vi "Process Helper.vi"(7 "UI Ref":refnum<vi>, 10 "current time":timestamp, 11 "Settings in":T1) -> (0 "Digital Values to Write":bool[](array[boolean]), 1 "Analog Values to Write":dbl[](array[numeric]), 2 "Sequence State Channels to Write":dbl[](array[numeric]), 3 "Settings out":T1, 4 "New Settings":string, 5 "Changed":bool)   [LabVIEW 2020, in "Sequencer with Output Values.lvlib" / "Sequencer with Output Values.lvclass"]
uses:
  Sequencer with Output Values.lvclass
  Params.ctl
  Step Settings.ctl
  <vilib>/FlexLogger/SDK/PluginSDK.lvlibp
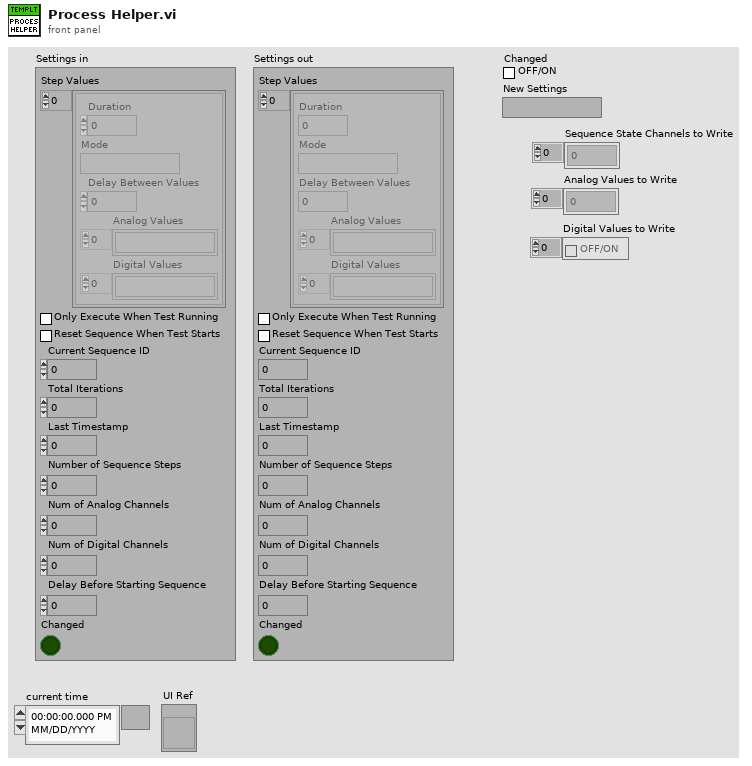
[diagram p1: front panel]
types:
  T1 = typedef "Sequencer with Output Values.lvlib/Sequencer with Output Values.lvclass/Params.ctl" = cluster{"Step Values":T2[], "Only Execute When Test Running":bool, "Reset Sequence When Test Starts":bool, "Current Sequence ID":u32, "Total Iterations":u32, "Last Timestamp":dbl, "Number of Sequence Steps":i32, "Num of Analog Channels":i32, "Num of Digital Channels":i32, "Delay Before Starting Sequence":dbl, "Changed":bool}
  T2 = typedef "Sequencer with Output Values.lvlib/Sequencer with Output Values.lvclass/Step Settings.ctl" = cluster{"Duration":dbl, "Mode":string, "Delay Between Values":dbl, "Analog Values":string[], "Digital Values":string[]}
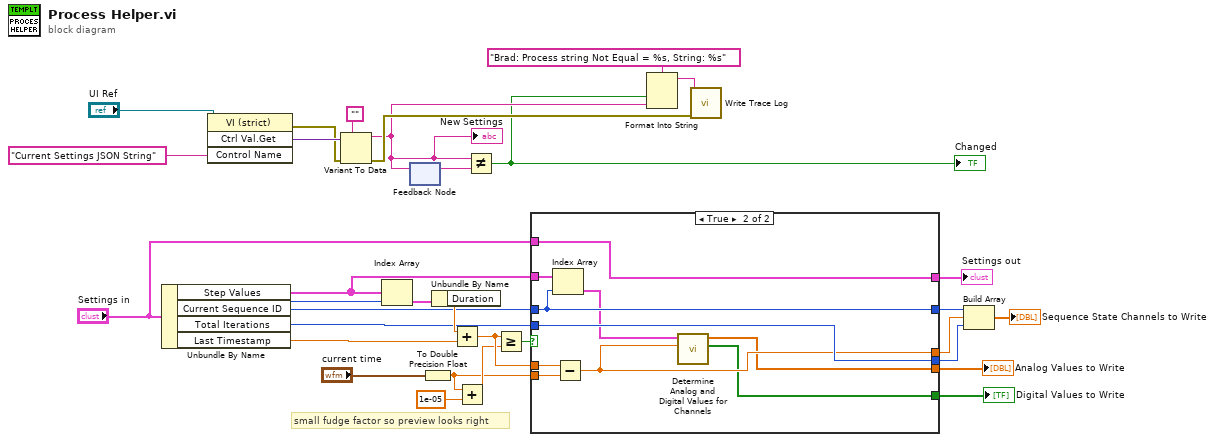
[diagram p0: block diagram]
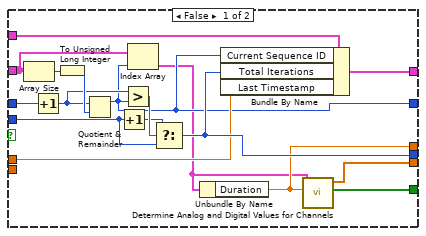
[diagram p2: hidden frame]
diagram:
  # "small fudge factor so preview looks right"
  n1 = Unbundle By Name("Settings in") -> ("Step Values"=w19:T2[], "Current Sequence ID"=w21:u32, "Total Iterations"=w20:u32, "Last Timestamp"=w23:dbl)
  n2 = invoke class="VI (strict)" method="Ctrl Val.Get"(reference="UI Ref", "Control Name"="Current Settings JSON String") -> (error out=w9:errorcluster, "Get Control Value Variant"=w10:variant)  [unwired: 2 in, 2 out]
  n3 = Variant To Data(error in=w9, type="", Variant=w10) -> (data=w4:string, error out=w5:errorcluster)
  "New Settings" <- w4
  n4 = Index Array(array=w19, index=w21) -> (element=w30:T2)
  n5 = feedback-in #1(w4) -> ()
  n6 = feedback #1() -> (w7:string)  [unwired: 1 in]
  n7 = To Double Precision Float(number="current time") -> (double precision float=w13:dbl)
  n8 = Unbundle By Name(w30) -> ("Duration"=w25:dbl)
  n9 = Add(x=w25, y=w23) -> (x+y=w27:dbl)
  n10 = Add(x=w13, y=1e-05) -> (x+y=w14:dbl)
  n11 = Not Equal?(x=w4, y=w7) -> (x != y?=w2:bool)
  "Changed" <- w2
  n12 = Greater Or Equal?(x=w27, y=w14) -> (x >= y?=w22:bool)
  n13 = case shown="True" w22 {
    tunnel: "Settings in" -> [w43 w57]
    tunnel: w21 -> [w47 w53]
    tunnel: w19 -> [w37 w54]
    tunnel: w20 -> [w45 w58]
    tunnel: [w36 w53] -> w24
    tunnel: [w41 w58] -> w26
    tunnel: [w42 w57] -> w31
    tunnel: w27 -> [w38 w56]
    tunnel: w13 -> [_ w55]
    tunnel: [w33 w51] -> w28
    tunnel: [w35 w50] -> w17
    tunnel: [w34 w49] -> w29
    frame False {
      n14 = Array Size(array=w37) -> (size(s)=w48:i32)
      n15 = Increment(x=w47) -> (x+1=w39:u32)
      n16 = To Unsigned Long Integer(number=w48) -> (unsigned 32bit integer=w40:u32)
      n17 = Quotient & Remainder(x=w39, y=w40) -> (x-y*floor(x/y)=w36:u32)  [unwired: 1 out]
      n18 = Increment(x=w45) -> (x+1=w44:u32)
      n19 = Greater?(x=w39, y=w36) -> (0:w46:bool)
      n20 = Index Array(array=w37, index=w36) -> (element=w32:T2)
      n21 = Select(t=w44, s=w46, f=w45) -> (s? t:f=w41:u32)
      n22 = Unbundle By Name(w32) -> ("Duration"=w33:dbl)
      n23 = Bundle By Name(cluster=w43, "Current Sequence ID"=w36, "Total Iterations"=w41, "Last Timestamp"=w38) -> (w42:T1)
      n24 = call "Determine Analog and Digital Values for Channels.vi"("Remaining Time"=w33, "Step Settings"=w32) -> ("Digital Values to Write"=w34:bool[], "Analog Values to Write"=w35:dbl[])  [unwired: 8 in]
    }
    frame True {
      n25 = Index Array(array=w54, index=w53) -> (element=w52:T2)
      n26 = Subtract(x=w56, y=w55) -> (x-y=w51:dbl)
      n27 = call "Determine Analog and Digital Values for Channels.vi"("Remaining Time"=w51, "Step Settings"=w52) -> ("Digital Values to Write"=w49:bool[], "Analog Values to Write"=w50:dbl[])  [unwired: 8 in]
    }
  }
  "Settings out" <- w31
  "Digital Values to Write" <- w29
  "Analog Values to Write" <- w17
  n28 = Format Into String(format string="Brad: Process string Not Equal = %s, String: %s", w2, w4) -> (resulting string=w6:string)  [unwired: 2 in, 1 out]
  n29 = call <vilib>:"Write Trace Log.vi"("error in (no error)"=w5, "Message"=w6) -> ()  [unwired: 9 in, 1 out]
  n30 = Build Array(w24, w28, w26) -> (→"Sequence State Channels to Write":dbl[])
